vi "Op-Graphics-Marker.vi"(6 "position":dbl format="%^.4e", 7 "marker interpolate":bool, 8 "error in (no error)":errorcluster, 9 "axis":i32(slide) scale=0.0..2.0, 10 "marker function":i32(slide) max=6 scale=0.0..6.0, 11 "VISA session":refnum<visa-resource-name>) -> (0 "error out":errorcluster, 3 "VISA resource name out":refnum<visa-resource-name>)   [LabVIEW 2016, in "Agilent 415X Series.lvlib"]
doc: "This VI controls the marker for GRAPHICS display. Executing this VI automatically switches the display mode to GRAPHICS."
uses:
  Agilent 415X Series.lvlib
panel:
  # "This VI will change the display mode to GRAPHICS"
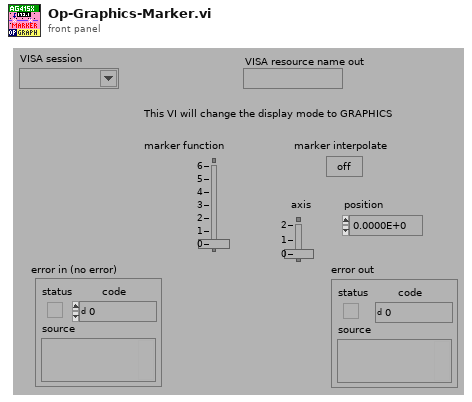
[diagram p1: front panel]
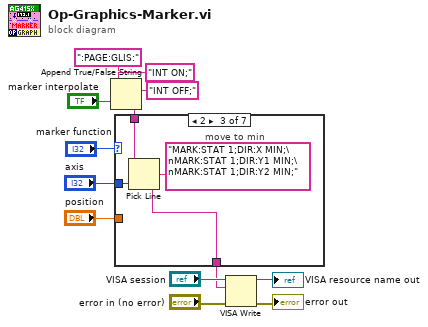
[diagram p0: block diagram]
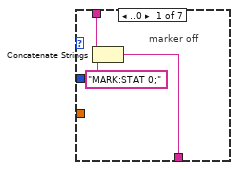
[diagram p2: hidden frame]
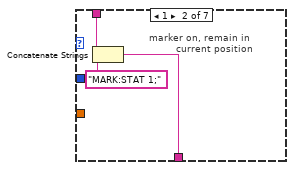
[diagram p3: hidden frame]
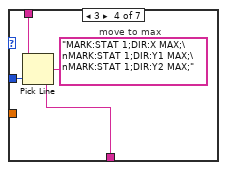
[diagram p4: hidden frame]
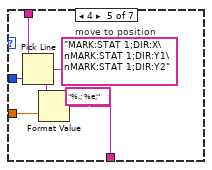
[diagram p5: hidden frame]
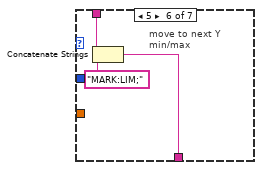
[diagram p6: hidden frame]
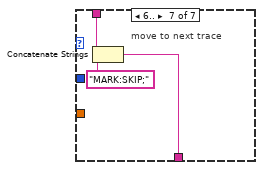
[diagram p7: hidden frame]
diagram:
  n1 = Append True/False String(1:"marker interpolate", 2:"INT OFF;", 3:"INT ON;", 4:":PAGE:GLIS:") -> (0:w6:string)
  n2 = case shown="2" "marker function" {
    tunnel: w6 -> [w16 w19 w22 w26 w33 w37 w40]
    tunnel: [w14 w17 w20 w24 w28 w35 w38] -> w2
    tunnel: "axis" -> [_ _ w23 w27 w34 _ _]
    tunnel: "position" -> [_ _ _ _ w29 _ _]
    frame ..0 {
      # "marker off"
      n3 = Concatenate Strings(w16, "MARK:STAT 0;") -> (w14:string)
    }
    frame 1 {
      # "marker on, remain in\n         current position"
      n4 = Concatenate Strings(w19, "MARK:STAT 1;") -> (w17:string)
    }
    frame 2 {
      # "move to min"
      n5 = Pick Line(string ("")=w22, multi-line string="MARK:STAT 1;DIR:X MIN;\nMARK:STAT 1;DIR:Y1 MIN;\nMARK:STAT 1;DIR:Y2 MIN;", line index=w23) -> (output string=w20:string)
    }
    frame 3 {
      # "move to max"
      n6 = Pick Line(string ("")=w26, multi-line string="MARK:STAT 1;DIR:X MAX;\nMARK:STAT 1;DIR:Y1 MAX;\nMARK:STAT 1;DIR:Y2 MAX;", line index=w27) -> (output string=w24:string)
    }
    frame 4 {
      # "move to position"
      n7 = Pick Line(string ("")=w33, multi-line string="MARK:STAT 1;DIR:X\nMARK:STAT 1;DIR:Y1\nMARK:STAT 1;DIR:Y2", line index=w34) -> (output string=w31:string)
      n8 = Format Value(string ("")=w31, format string="%.; %e;", value (0)=w29) -> (output string=w28:string)
    }
    frame 5 {
      # "move to next Y\nmin/max"
      n9 = Concatenate Strings(w37, "MARK:LIM;") -> (w35:string)
    }
    frame 6.. {
      # "move to next trace"
      n10 = Concatenate Strings(w40, "MARK:SKIP;") -> (w38:string)
    }
  }
  n11 = VISA Write(VISA resource name="VISA session", write buffer=w2, error in (no error)="error in (no error)") -> (VISA resource name out=→"VISA resource name out":refnum<visa-resource-name>, error out=→"error out":errorcluster)  [unwired: 1 out]
